vi "Write to File.vi"(8 "error in (no error)":errorcluster, 10 "INI Ref":T1, 11 "Action Step in":refnum<class "Action Step.lvclass">) -> (0 "error out":errorcluster, 2 "INI Ref out":T1, 3 "Action Step out":refnum<class "Action Step.lvclass">)   [LabVIEW 2020, in "MacroAssert.lvlib" / "Action Step.lvclass"]
uses:
  Action Step.lvclass
  C:/Users/acasalen/Documents/LabVIEW Data/Projects/MacroAssert/source/Classes/Step/Step.lvclass
  <vilib>/Utility/config.llb/Config Data RefNum.ctl
  <vilib>/Utility/config.llb/Write Key (I32).vi
  Step/Step.lvclass
  MacroAssert.lvlib
  <vilib>/Utility/config.llb/NI_LVConfig.lvlib
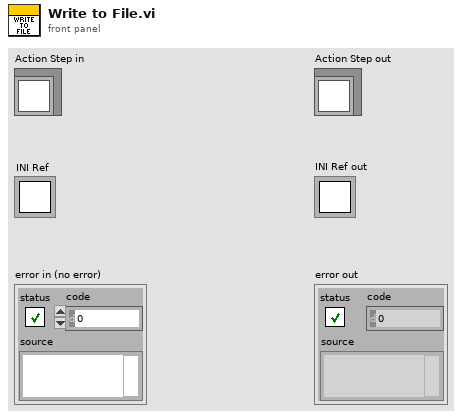
[diagram p1: front panel]
types:
  T1 = typedef "NI_LVConfig.lvlib/Config Data RefNum.ctl" = refnum<k1>
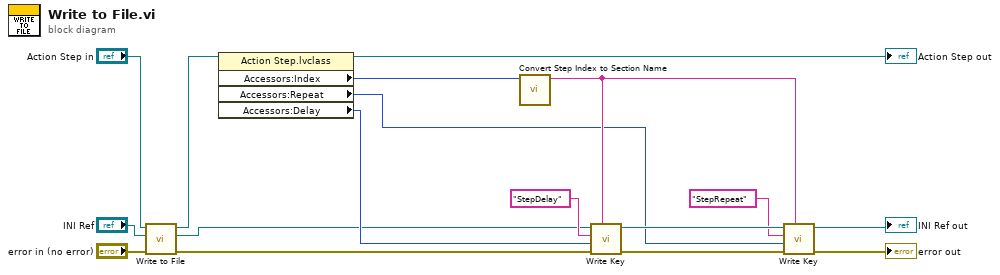
[diagram p0: block diagram]
diagram:
  n1 = call-parent "Write to File.vi"("error in (no error)"="error in (no error)", "INI Ref"="INI Ref", "Step in"="Action Step in") -> ("error out"=w6:errorcluster, "INI Ref out"=w1:T1, "Step out"=w4:refnum<class "Action Step.lvclass">)  [unwired: 6 in]
  n2 = property class="Action Step.lvclass"(reference=w4) -> (reference out=→"Action Step out":refnum<class "Action Step.lvclass">, "Accessors:Index"=w10:i32, "Accessors:Repeat"=w7:i32, "Accessors:Delay"=w8:i32)  [unwired: 1 in, 1 out]
  n3 = call "Convert Step Index to Section Name.vi"("Step Index"=w10) -> ("Section Name"=w9:string)  [unwired: 10 in]
  n4 = call-poly <vilib>:"Write Key.vi"("section"=w9, "error in (no error)"=w6, "value"=w8, "key"="StepDelay", "refnum"=w1) -> ("error out"=w12:errorcluster, "refnum out"=w14:T1)  [unwired: 4 in, 1 out]
  n5 = call-poly <vilib>:"Write Key.vi"("section"=w9, "error in (no error)"=w12, "value"=w7, "key"="StepRepeat", "refnum"=w14) -> ("error out"=→"error out":errorcluster, "refnum out"=→"INI Ref out":T1)  [unwired: 4 in, 1 out]
